vi "HRTF-Build Filename.vi"(0 "State":T2, 7 "Mic":T1) -> (4 "path":path, 8 "filestem":string)   [LabVIEW 2015]
uses:
  Typedefs/HRTF-State.ctl
  Typedefs/HRTF-Laterality.ctl
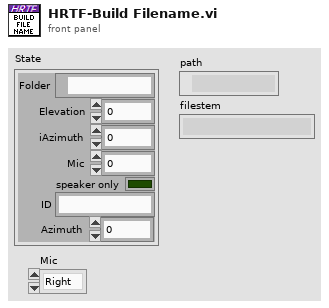
[diagram p1: front panel]
types:
  T1 = typedef "HRTF-Laterality.ctl" = enum16{"Right", "Left"}
  T2 = typedef "HRTF-State.ctl" = cluster{"Folder":path, "Elevation":dbl, "iAzimuth":i32, "Mic":i32, "speaker only":bool, "ID":string, "Azimuth":dbl}
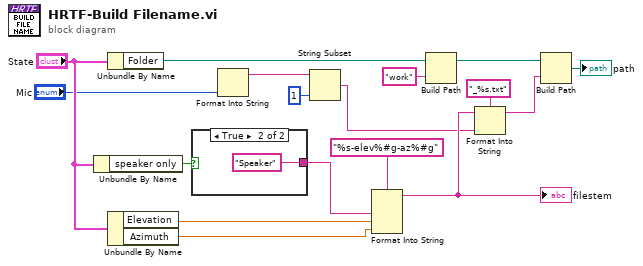
[diagram p0: block diagram]
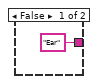
[diagram p2: hidden frame]
diagram:
  n1 = Unbundle By Name("State") -> ("speaker only"=w16:bool)
  n2 = Unbundle By Name("State") -> ("Folder"=w13:path)
  n3 = Unbundle By Name("State") -> ("Elevation"=w2:dbl, "Azimuth"=w1:dbl)
  n4 = case shown="True" w16 {
    tunnel: ["Ear" "Speaker"] -> w14
    frame False {
    }
    frame True {
    }
  }
  n5 = Format Into String("Mic") -> (resulting string=w7:string)  [unwired: 3 in, 1 out]
  n6 = String Subset(string=w7, length (rest)=1 ("length (rest)")) -> (substring=w5:string)  [unwired: 1 in]
  n7 = Format Into String(format string="%s-elev%#g-az%#g", w14, w2, w1) -> (resulting string=w11:string)  [unwired: 2 in, 1 out]
  "filestem" <- w11
  n8 = Build Path(base path=w13, name or relative path="work") -> (appended path=w4:path)
  n9 = Format Into String(format string="_%s.txt", initial string=w11, w5) -> (resulting string=w10:string)  [unwired: 1 in, 1 out]
  n10 = Build Path(base path=w4, name or relative path=w10) -> (appended path=→"path":path)
